vi "Configure Data Interleave.vi"(6 "Data Interleave (1)":i32=1, 7 "Channel (1: Channel 1)":i32(ring)=1 items=["All"=0, "Channel 1"=1, "Channel 1.1"=11, "Channel 1.2"=12, "Channel 1.3"=13, "Channel 1.4"=14, "Channel 2"=2, "Channel 2.1"=21, "Channel 2.2"=22, "Channel 2.3"=23, "Channel 2.4"=24, "Channel 3"=3, "Channel 3.1"=31, "Channel 3.2"=32, "Channel 3.3"=33, "Channel 3.4"=34, "Channel 4"=4, "Channel 4.1"=41, "Channel 4.2"=42, "Channel 4.3"=43, "Channel 4.4"=44], 8 "error in (no error)":errorcluster, 9 "Number of Averages (1)":i32=1, 10 "Sensor Number (1)":i32=1, 11 "VISA resource name":refnum<visa-resource-name>) -> (0 "error out":errorcluster, 3 "VISA resource name out":refnum<visa-resource-name>)   [LabVIEW 2015, in "Micron Optics sm130.lvlib"]
doc: "Configures data interleave and number of averages to specified channel and sensor. \n\n<b>Note:</b>\nBy using data interleave, the instrument continues to acquire data at its full rate while only reporting data at a reduced rate as determined by Data Interleave Parameter. Asthe module continues to acquire at max rate, data is available between periods of reporting to facilitate averaging. Averaging reduces the noise of the measurement."
uses:
  Micron Optics sm130.lvlib
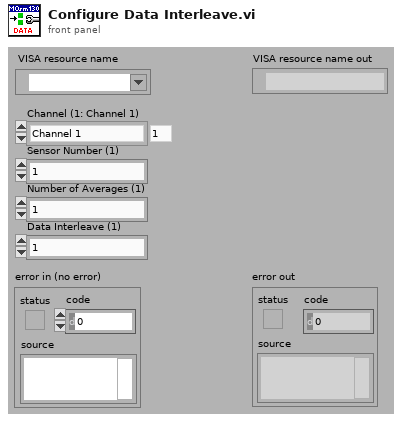
[diagram p1: front panel]
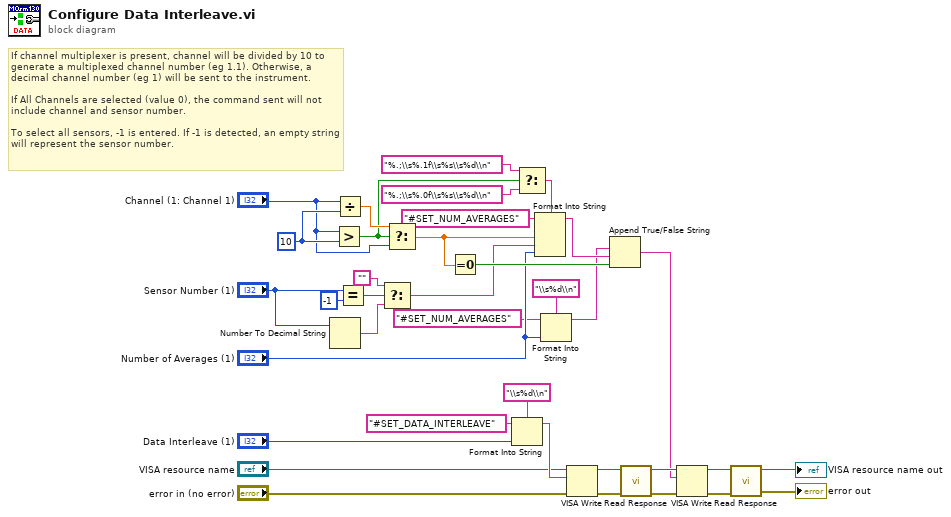
[diagram p0: block diagram]
diagram:
  w35 = 10 ("y")
  # "If channel multiplexer is present, channel will be divided by 10 to generate a multiplexed channel number (eg 1.1). Otherwise, a decimal channel number (eg 1) will be sent to the instrument.\n\nIf All Channels are selected (value 0), the command sent will not include channel and sensor number. \n \nTo select all sensors, -1 is entered. If -1 is detected, an empty string will represent the sensor number."
  n1 = Number To Decimal String(number="Sensor Number (1)") -> (decimal integer string=w23:string)  [unwired: 1 in]
  n2 = Greater?(x="Channel (1: Channel 1)", y=w35) -> (0:w34:bool)
  n3 = Divide(x="Channel (1: Channel 1)", y=w35) -> (x/y=w36:dbl)
  n4 = Equal?(x="Sensor Number (1)", y=-1) -> (x = y?=w25:bool)
  n5 = Select(t="", s=w25, f=w23) -> (s? t:f=w21:string)
  n6 = Select(t=w36, s=w34, f="Channel (1: Channel 1)") -> (s? t:f=w30:dbl)
  n7 = Equal To 0?(x=w30) -> (x = 0?=w28:bool)
  n8 = Format Into String(format string="\\s%d\\n", initial string="#SET_DATA_INTERLEAVE", "Data Interleave (1)") -> (resulting string=w11:string)  [unwired: 1 in, 1 out]
  n9 = Select(t="%.;\\s%.1f\\s%s\\s%d\\n" ("format string"), s=w34, f="%.;\\s%.0f\\s%s\\s%d\\n" ("format string")) -> (s? t:f=w31:string)
  n10 = Format Into String(format string=w31, initial string="#SET_NUM_AVERAGES", w30, w21, "Number of Averages (1)") -> (resulting string=w29:string)  [unwired: 1 in, 1 out]
  n11 = Format Into String(format string="\\s%d\\n", initial string="#SET_NUM_AVERAGES", "Number of Averages (1)") -> (resulting string=w17:string)  [unwired: 1 in, 1 out]
  n12 = VISA Write(VISA resource name="VISA resource name", write buffer=w11, error in (no error)="error in (no error)") -> (VISA resource name out=w13:refnum<visa-resource-name>, error out=w12:errorcluster)  [unwired: 1 out]
  n13 = Append True/False String(1:w28, 2:w29, 3:w17) -> (0:w5:string)  [unwired: 1 in]
  n14 = call "Read Response.vi"("error in (no error)"=w12, "VISA resource name"=w13) -> ("error out"=w7:errorcluster, "VISA resource name out"=w6:refnum<visa-resource-name>)  [unwired: 7 in, 1 out]
  n15 = VISA Write(VISA resource name=w6, write buffer=w5, error in (no error)=w7) -> (VISA resource name out=w8:refnum<visa-resource-name>, error out=w9:errorcluster)  [unwired: 1 out]
  n16 = call "Read Response.vi"("error in (no error)"=w9, "VISA resource name"=w8) -> ("error out"=→"error out":errorcluster, "VISA resource name out"=→"VISA resource name out":refnum<visa-resource-name>)  [unwired: 7 in, 1 out]
